vi "Tool Q LEIN solonoid  two valves task.vi"(0 "outpuyt channel1":u8, 5 "current limit(0.2A)":dbl, 7 "outpuyt channel2":u8, 9 "time (50 ms)":u16, 11 "error in (no error)":errorcluster) -> (4 "LEIN custom reply Q":T1, 15 "error out":errorcluster)   [LabVIEW 2011]
uses:
  LEINmaster/Defenitions/LEIN custom reply Q.ctl
  LEINmaster/Defenitions/LEIN Reply Holder.ctl
  LEINmaster/Defenitions/LEIN CMD Cluster.ctl
  LEINmaster/Defenitions/LEIN CMD List.ctl
  LEINmaster/Defenitions/LEIN Structure variations.ctl
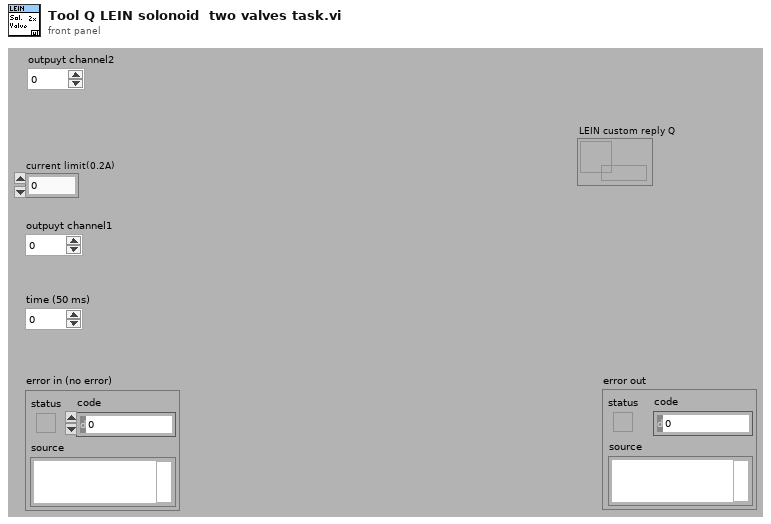
[diagram p1: front panel]
types:
  T1 = typedef "LEIN custom reply Q.ctl" = refnum<queue>
  T2 = typedef "LEIN Structure variations.ctl" = enum16{"LEIN08", "LEIN31", "LEIN63"}
  T3 = enum16{"big-endian, network order", "native, host order", "little-endian"}
  T4 = typedef "LEIN CMD Cluster.ctl" = cluster{"SID":u8, "ANF":bool, "CMD":T5, "DATA":u8[]}
  T5 = typedef "LEIN CMD List.ctl" = enum8{"ACTI", "TASK", "RES0", "STAT", "RES1", "RES2", "RES3", "USER"}
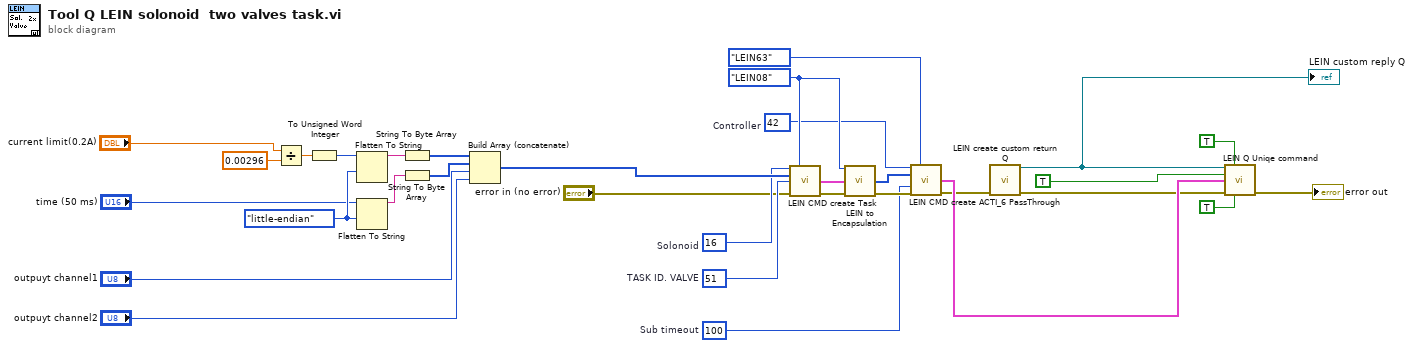
[diagram p0: block diagram]
diagram:
  w10 = u8 42  # Controller
  w11 = u8 16  # Solonoid
  w17 = u16 100  # Sub timeout
  w14 = u8 51  # TASK ID. VALVE
  w13 = LEIN_Structure_variations."LEIN08" ("LEIN Variation")
  w26 = T3."little-endian" ("byte order (0:big-endian, network order)")
  n1 = Divide(x="current limit(0.2A)", y=0.00296 ("x")) -> (x/y=w31:dbl)
  n2 = To Unsigned Word Integer(number=w31) -> (unsigned 16bit integer=w29:u16)
  n3 = Flatten To String(anything=w29, byte order (0:big-endian, network order)=w26) -> (data string=w28:string)  [unwired: 2 in, 2 out]
  n4 = Flatten To String(anything="time (50 ms)", byte order (0:big-endian, network order)=w26) -> (data string=w24:string)  [unwired: 2 in, 2 out]
  n5 = String To Byte Array(string=w28) -> (unsigned byte array=w27:u8[])
  n6 = String To Byte Array(string=w24) -> (unsigned byte array=w23:u8[])
  n7 = Build Array (concatenate)(w27, w23, "outpuyt channel1", "outpuyt channel2") -> (w12:u8[])
  n8 = call "LEIN CMD create Task.vi"("SID"=w11, "LEIN Variation"=w13, "Data"=w12, "TASK ID"=w14, "error in (no error)"="error in (no error)") -> ("CMD"=w15:T4, "error out"=w16:errorcluster)  [unwired: 9 in]
  n9 = call "LEIN to Encapsulation.vi"("LEIN Variation"=w13, "CMD"=w15, "error in (no error)"=w16) -> ("Data and header"=w18:u8[], "error out"=w19:errorcluster)  [unwired: 8 in, 3 out]
  n10 = call "LEIN CMD create ACTI_6 PassThrough.vi"("SID"=w10, "LEIN Variation"=LEIN_Structure_variations."LEIN63", "LEIN ecapsulated data (header and data)"=w18, "Sub Timeout (ms)"=w17, "error in (no error)"=w19) -> ("CMD"=w6:T4, "error out"=w5:errorcluster)  [unwired: 9 in]
  n11 = call "LEIN create custom return Q.vi"("error in (no error)"=w5) -> ("LEIN custom reply Q"=w3:T1, "error out"=w4:errorcluster)  [unwired: 13 in]
  "LEIN custom reply Q" <- w3
  n12 = call "LEIN Q Uniqe command.vi"("LEIN custom reply Q"=w3, "Retry on err (F)"=TRUE, "Custom Q(F)"=TRUE, "CMD"=w6, "error in"=w4, "priority(F)"=TRUE) -> ("error out"=→"error out":errorcluster)  [unwired: 9 in]
